vi "DN4_DI_DetectInterrupt.vi"(9 "error in (no error)":errorcluster, 10 "status":bool, 11 "Task ID":u32) -> (0 "error out":errorcluster, 1 "interrupt source":i32, 2 "snap data":u8[](array[numeric]), 3 "Task out ID":u32)   [LabVIEW 2009]
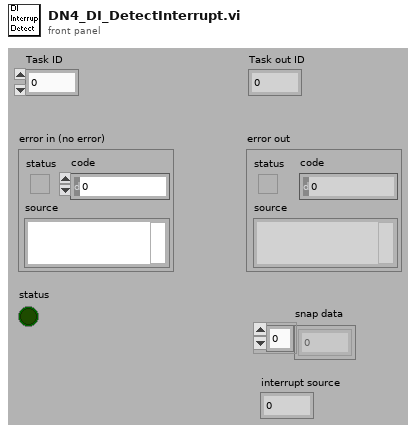
[diagram p1: front panel]
types:
  T1 = cluster{"interrupt source":i64, "port data":u8[]}
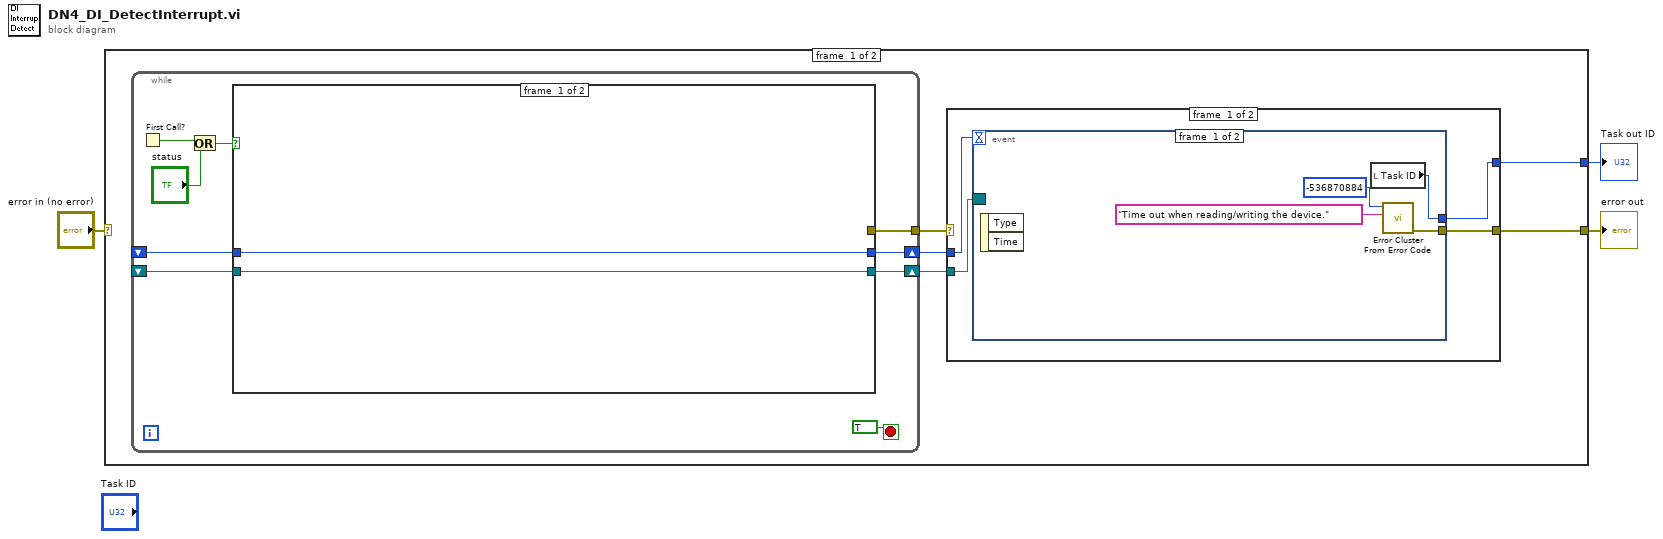
[diagram p0: block diagram]
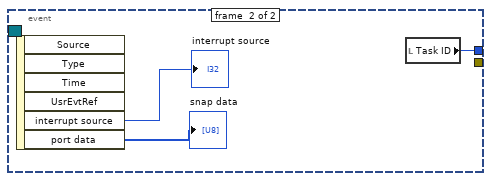
[diagram p2: hidden frame]
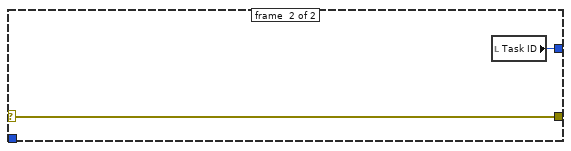
[diagram p3: hidden frame]
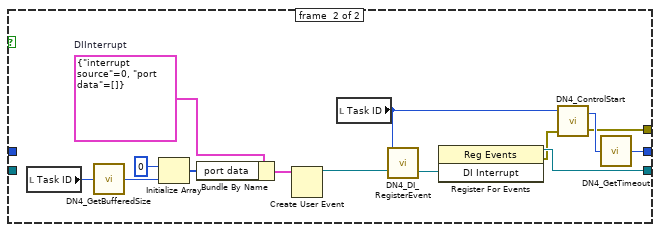
[diagram p4: hidden frame]
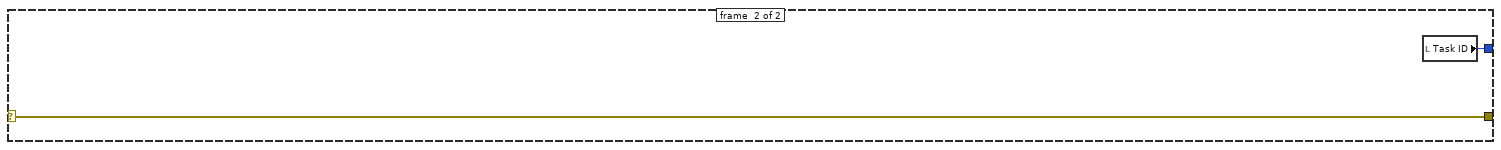
[diagram p5: hidden frame]
diagram:
  n1 = case shown="No Error" "error in (no error)" {
    selector: "error in (no error)" -> [_ w48]
    tunnel: [w6 w48] -> w2
    tunnel: [w5 w47] -> w1
    frame #0 {
      n2 = while {
        shift-right: [w27] -> w7
        shift-left: _ -> [w29]
        shift-right: [w28] -> w8
        shift-left: _ -> [w26]
        tunnel: [w25] -> w4
        stop <- TRUE stop-if-true
        n3 = First Call?() -> (First Call?: T/F=w24:bool)
        n4 = Or(x=w24, y="status") -> (x .or. y?=w22:bool)
        n5 = case shown="True" w22 {
          tunnel: [w32 w43] -> w27
          tunnel: w29 -> [w32 _]
          tunnel: [w31 w44] -> w28
          tunnel: w26 -> [w31 _]
          tunnel: [_ w42] -> w25
          frame #0 {
          }
          frame #1 {
            w39 = T1 {"interrupt source"=0, "port data"=[]}  # DIInterrupt
            n6 = local read "Task ID"() -> (w36:u32)
            n7 = call <userlib>:"DN4_GetBufferedSize.vi"("Task ID"=w36) -> ("return type"=w40:i32)
            n8 = Initialize Array(u8 0 ("element"), w40) -> (w37:u8[])
            n9 = Bundle By Name(cluster=w39, "port data"=w37) -> (w35:T1)
            n10 = Create User Event(user event datatype=w35) -> (user event=w34:refnum<user-event>)  [unwired: 1 in, 1 out]
            n11 = local read "Task ID"() -> (w46:u32)
            n12 = call <userlib>:"DN4_DI_RegisterEvent.vi"("DI Interrupt"=w34, "Task ID"=w46) -> ("DI Interrupt"=w33:refnum<user-event>)  [unwired: 1 out]
            n13 = register-events(w33) -> (reference out=w43:refnum<event-registration>, error out=w41:errorcluster)  [unwired: 2 in]
            n14 = call <userlib>:"DN4_ControlStart.vi"("error in (no error)"=w41, "Task ID"=w46) -> ("error out"=w42:errorcluster, "Task ID"=w45:u32)  [unwired: 1 out]
            n15 = call <userlib>:"DN4_GetTimeout.vi"("Task ID"=w45) -> ("return type"=w44:i32)
          }
        }
      }
      n16 = case shown="No Error" w4 {
        selector: w4 -> [_ w21]
        tunnel: w8 -> [w12 _]
        tunnel: w7 -> [w11 _]
        tunnel: [w10 w21] -> w6
        tunnel: [w9 w20] -> w5
        frame #0 {
          n17 = event shown="[1] <DI Interrupt>: User Event" {
            selector: w11 -> [_ _]
            dyn-events: _ -> [_ _]
            timeout: w12 -> [_ _]
            tunnel: [w14 _] -> w10
            tunnel: [w13 w19] -> w9
            event #0 {
              n18 = event-data() -> ()  [unwired: 3 out]
              n19 = local read "Task ID"() -> (w13:u32)
              n20 = call <vilib>:"Error Cluster From Error Code.vi"("error message (\"\")"="Time out when reading/writing the device." ("error message (\"\")"), "error code (0)"=-536870884) -> ("error out"=w14:errorcluster)  [unwired: 2 in, 5 out]
            }
            event #1 {
              n21 = event-data() -> ("interrupt source"=→"interrupt source":i64, "port data"=→"snap data":u8[])  [unwired: 5 out]
              n22 = local read "Task ID"() -> (w19:u32)
            }
          }
        }
        frame #1 {
          n23 = local read "Task ID"() -> (w20:u32)
        }
      }
    }
    frame #1 {
      n24 = local read "Task ID"() -> (w47:u32)
    }
  }
  "error out" <- w2
  "Task out ID" <- w1
